vi "Robot Information Global.vi"() -> ()   [LabVIEW 2018]
panel:
  in  "What Auton?":T1(ring)
  in  "Robot Size":cluster{"Robot Width":dbl, "Robot Length":dbl}={"Robot Width"=21.5, "Robot Length"=25.5}
  in  "Cargo State":enum16{""}(ring)
  in  "Hatch Pannel State":enum16{""}(ring)
  in  "Lift State":enum16{""}(ring)
  in  "HAB Climber State":enum16{""}(ring)
  in  "Practice Robot":bool
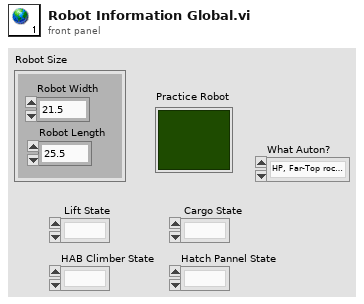
[diagram p1: front panel]
types:
  T1 = enum16{"HP, Far-Top rocket, Lvl2 Right", "HP, Far-Top rocket, Lvl2 Left", "HP, Far-Top rocket, Lvl1 Right", "HP, Far-Top rocket, Lvl1 Left", "HP, Both-Top rocket, Lvl2 Right", "HP, Both-Top rocket, Lvl2 Left", "HP, Both-Top rocket, Lvl1 Right", "HP, Both-Top rocket, Lvl1 Left", "HP, Near cargo, Lvl2 ", "HP, Near cargo, Lvl1", "HP, Far cargo, Lvl2 ", "HP, Far cargo, Lvl1"}
diagram:
